vi "remove channel from active arrayv2.vi"(0 "line array in":u32[](array[numeric]), 1 "line to remove":u32) -> (2 "line array out":u32[](array[numeric]), 3 "removal":bool, 4 "index":i32)   [LabVIEW 2015]
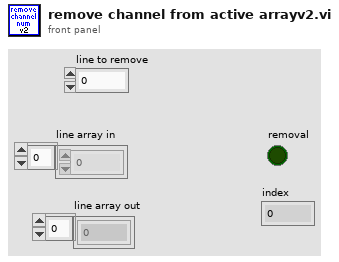
[diagram p1: front panel]
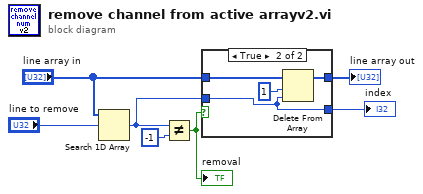
[diagram p0: block diagram]
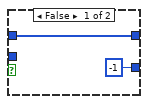
[diagram p2: hidden frame]
diagram:
  n1 = Search 1D Array(1D array="line array in", element="line to remove") -> (index of element=w2:i32)  [unwired: 1 in]
  n2 = Not Equal?(x=w2, y=-1) -> (x != y?=w3:bool)
  "removal" <- w3
  n3 = case shown="True" w3 {
    tunnel: "line array in" -> [w9 w13]
    tunnel: [w9 w11] -> w7
    tunnel: w2 -> [_ w10]
    tunnel: [-1 ("index of element") w10] -> w1
    frame False {
    }
    frame True {
      n4 = Delete From Array(array=w13, length=1, index=w10) -> (array with subset deleted=w11:u32[])  [unwired: 1 out]
    }
  }
  "line array out" <- w7
  "index" <- w1
